vi "PH_ImageCalibrator.save calibration data.vi"(0 "i ref in":refnum<vi>, 5 "error in (no error)":errorcluster) -> (14 "i ref out":refnum<vi>, 19 "error out":errorcluster)   [LabVIEW 2014, in "PH_ImageCalibrator.lvlib"]
doc: "This VI saves the calibration data."
uses:
  PH_ImageCalibrator.lvlib
  PH_ImageCalibrator.Calibration Data.ctl
  PH_Img_BaseClass/PH_Img_BaseClass.lvlib
panel:
  in  "Calibration data":T1
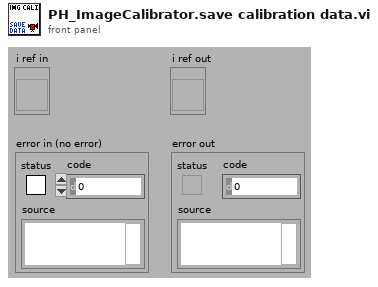
[diagram p1: front panel]
types:
  T1 = typedef "PH_ImageCalibrator.lvlib/PH_ImageCalibrator.Calibration Data.ctl" = cluster{"Date":string, "Time":string, "Cam Settings":cluster{"Cam ID":string, "Gain":dbl, "Brightness":dbl, "Shutter":dbl, "Cam Error":bool, "Mode":i32}, "Background Image":cluster{"Image":dbl[][], "Image Error":bool}, "Linear Calibration":cluster{"Calibration Factor":dbl, "not mm or mrad":bool}, "Energy Calibration":cluster{"Calibration Factor":dbl, "no mJ":bool}}
  T2 = typedef "PH_ImageCalibrator.lvlib/PH_ImageCalibrator.i attribute.ctl" = cluster{"GUI Refs":cluster{"Available Cams":refnum<vi>, "OK":refnum<vi>, "Skip":refnum<vi>, "Repeat":refnum<vi>, "Cancel":refnum<vi>, "Length [mm]":refnum<vi>, "Energy [mJ]":refnum<vi>, "Dialog":refnum<vi>}, "Cam instances":string[], "Dark Pics":cluster{"#":i32, "BI taken":bool}, "Lin Cali":cluster{"Distance [Pixel]":dbl, "Distance [mm]":dbl, "Lin Cali Factor [mm/Pixel]":dbl}, "Energy Cali":cluster{"Pixelsum":dbl, "Energy [mJ]":dbl, "Energy Cali factor [mJ/Pixelsum]":dbl, "Underground subtracted?":bool, "#":i32}, "Images":cluster{"Background":T3, "Energy":T3}}
  T3 = typedef "IMAQ Image.ctl" = refnum<image>
  T4 = typedef "PH_Img_BaseClass.lvlib/PH_Img_BaseClass.i attribute.ctl" = cluster{"GUI Refs":T5, "Timeout Image [ms]":i32, "Default Periodic Period [ms]":i32, "Camera":cluster{"Instancename":string, "Notifier":refnum<notifier>}, "Palette":T6, "Cam Settings":cluster{"Cam ID":string, "Gain":dbl, "Brightness":dbl, "Shutter":dbl, "Cam Info Failure":bool, "Mode":i32}}
  T5 = typedef "PH_Img_BaseClass.lvlib/PH_Img_BaseClass.GUI Refs.ctl" = cluster{"Timeout":refnum<vi>, "Image":refnum<vi>, "Palette":refnum<vi>, "Timeout Set":refnum<vi>}
  T6 = typedef "PH_Img_BaseClass.lvlib/PH_Img_BaseClass.Palette.ctl" = i32
  T7 = cluster{"Cam ID":string, "Gain":dbl, "Brightness":dbl, "Shutter":dbl, "Cam Info Failure":bool, "Mode":i32}
  T8 = enum16{"open", "replace", "create", "open or create", "replace or create", "replace or create with confirmation"}
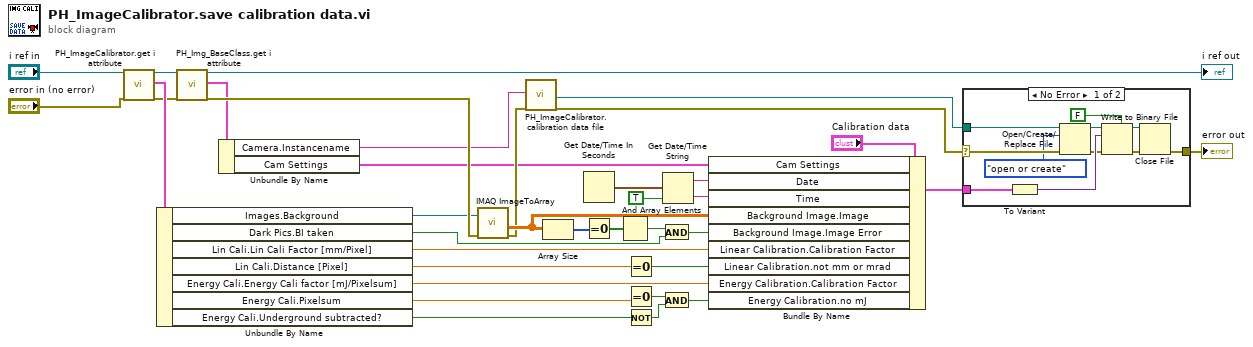
[diagram p0: block diagram]
diagram:
  n1 = call "PH_ImageCalibrator.get i attribute.vi"("i ref in"="i ref in", "error in (no error)"="error in (no error)") -> ("i ref out"=w6:refnum<vi>, "i attribute"=w34:T2, "error out"=w10:errorcluster)  [unwired: 15 in]
  n2 = Unbundle By Name(w34) -> ("Images.Background"=w1:T3, "Dark Pics.BI taken"=w13:bool, "Lin Cali.Lin Cali Factor [mm/Pixel]"=w25:dbl, "Lin Cali.Distance [Pixel]"=w24:dbl, "Energy Cali.Energy Cali factor [mJ/Pixelsum]"=w23:dbl, "Energy Cali.Pixelsum"=w22:dbl, "Energy Cali.Underground subtracted?"=w21:bool)
  n3 = call "PH_Img_BaseClass.get i attribute.vi"("i ref in"=w6, "error in (no error)"=w10) -> ("i ref out"=→"i ref out":refnum<vi>, "i attribute"=w4:T4, "error out"=w7:errorcluster)  [unwired: 15 in]
  n4 = Unbundle By Name(w4) -> ("Camera.Instancename"=w3:string, "Cam Settings"=w2:T7)
  n5 = call "IMAQ ImageToArray"("error in (no error)"=w7, "Image"=w1) -> ("Image Pixels (Float)"=w9:sgl[][], "error out"=w8:errorcluster)  [unwired: 2 in, 3 out]
  n6 = call "PH_ImageCalibrator.calibration data file.vi"("Camera Instance"=w3, "error in"=w8) -> ("File to save Cam Calibration Data in"=w17:path, "error out"=w11:errorcluster)  [unwired: 16 in]
  n7 = Array Size(array=w9) -> (size(s)=w28:i32[])
  n8 = Get Date/Time In Seconds() -> (seconds since 1Jan1904=w30:timestamp)
  n9 = Equal To 0?(x=w28) -> (x = 0?=w27:bool[])
  n10 = And Array Elements(Boolean array=w27) -> (logical AND=w14:bool)
  n11 = Equal To 0?(x=w24) -> (x = 0?=w26:bool)
  n12 = Equal To 0?(x=w22) -> (x = 0?=w19:bool)
  n13 = Not(x=w21) -> (.not. x?=w20:bool)
  n14 = And(x=w14, y=w13) -> (x .and. y?=w12:bool)
  n15 = And(x=w19, y=w20) -> (x .and. y?=w18:bool)
  n16 = Get Date/Time String(seconds (now)=w30, want seconds? (F)=TRUE) -> (date string=w32:string, time string=w31:string)  [unwired: 1 in]
  n17 = Bundle By Name(cluster="Calibration data", "Cam Settings"=w2, "Date"=w32, "Time"=w31, "Background Image.Image"=w9, "Background Image.Image Error"=w12, "Linear Calibration.Calibration Factor"=w25, "Linear Calibration.not mm or mrad"=w26, "Energy Calibration.Calibration Factor"=w23, "Energy Calibration.no mJ"=w18) -> (w16:T1)
  n18 = case shown="No Error" w11 {
    selector: w11 -> [w41 w48]
    tunnel: [w45 w48] -> w15
    tunnel: w17 -> [w39 _]
    tunnel: w16 -> [w43 _]
    frame No Error {
      n19 = To Variant(anything=w43) -> (Variant=w44:variant)
      n20 = Open/Create/Replace File(file path (use dialog)=w39, error in=w41, operation (0:open)=T8."open or create") -> (refnum out=w37:refnum<file>, error out=w40:errorcluster)  [unwired: 3 in, 1 out]
      n21 = Write to Binary File(file (use dialog)=w37, data=w44, error in=w40, 5:FALSE ("prepend array or string size? (T)")) -> (refnum out=w46:refnum<file>, error out=w47:errorcluster)  [unwired: 2 in, 1 out]
      n22 = Close File(refnum=w46, error in=w47) -> (error out=w45:errorcluster)  [unwired: 1 out]
    }
    frame Error {
    }
  }
  "error out" <- w15
